vi "服务器引用层次.vi"(1 "服务器引用层次 i":T1, 2 "模式":enum16{"读取", "写入"}(ring)) -> (0 "服务器引用层次 o":T1)   [LabVIEW 2013]
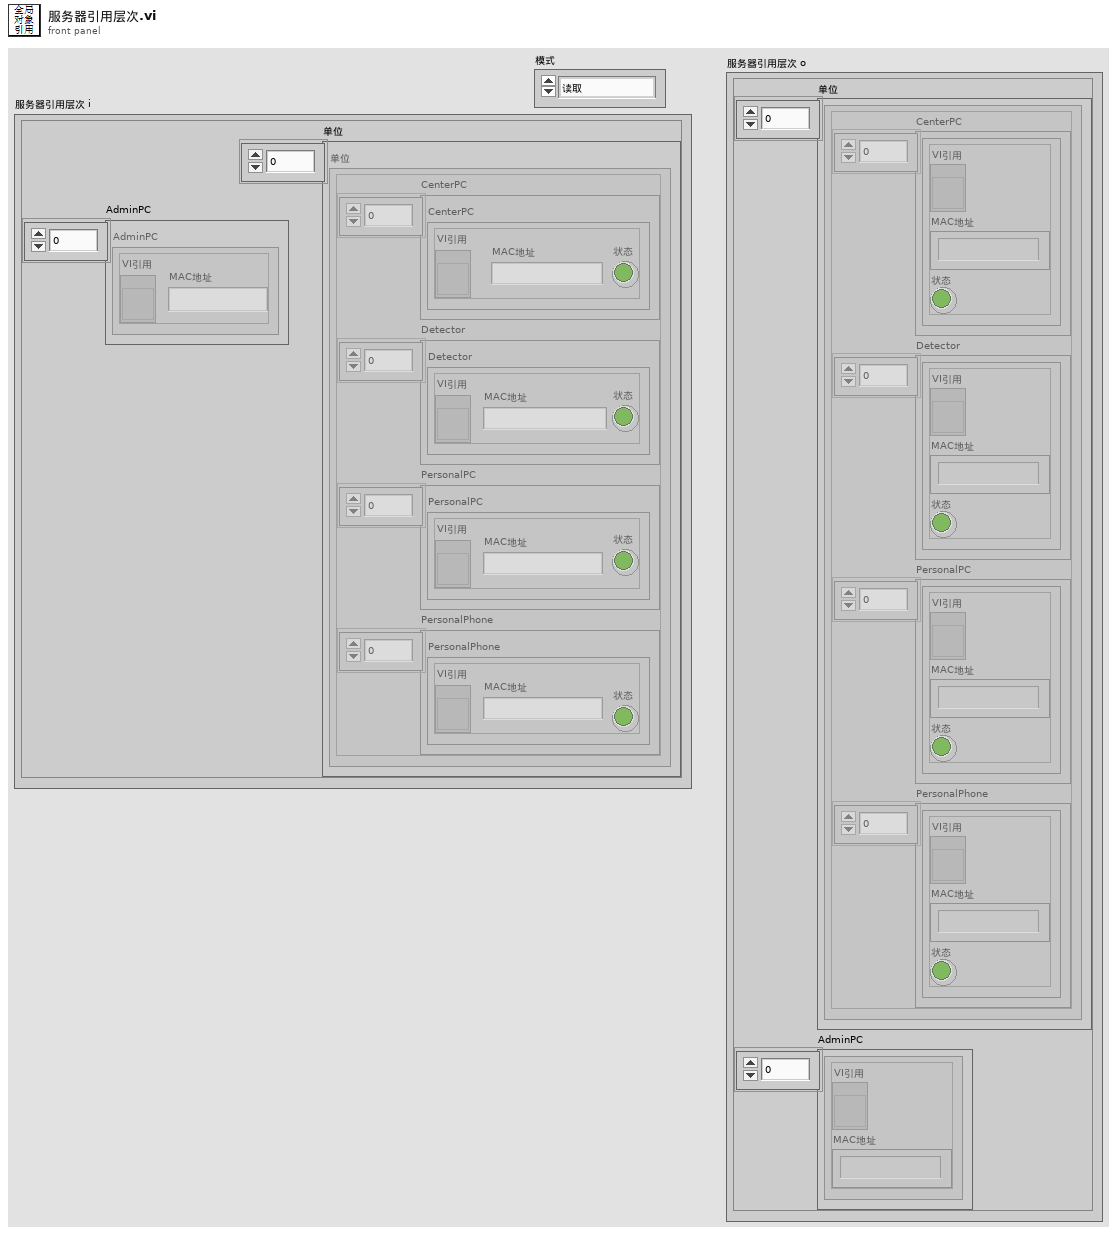
[diagram p1: front panel]
types:
  T1 = cluster{"单位":cluster{"CenterPC":cluster{"VI引用":refnum<vi>, "MAC地址":string, "状态":bool}[], "Detector":cluster{"VI引用":refnum<vi>, "MAC地址":string, "状态":bool}[], "PersonalPC":cluster{"VI引用":refnum<vi>, "MAC地址":string, "状态":bool}[], "PersonalPhone":cluster{"VI引用":refnum<vi>, "MAC地址":string, "状态":bool}[]}[], "AdminPC":cluster{"VI引用":refnum<vi>, "MAC地址":string}[]}
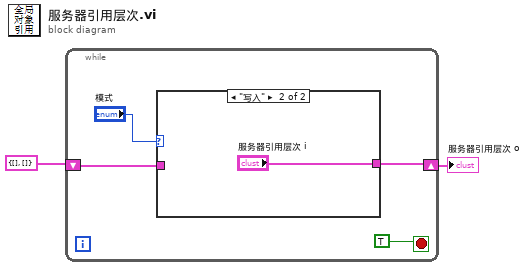
[diagram p0: block diagram]
diagram:
  n1 = while {
    shift-right: [w4] -> w1
    shift-left: T1 {"单位"=[], "AdminPC"=[]} ("服务器引用层次") -> [w3]
    stop <- TRUE stop-if-true
    n2 = case shown="\"写入\"" "模式" {
      tunnel: [w7 "服务器引用层次 i"] -> w4
      tunnel: w3 -> [w7 _]
      frame "读取", Default {
      }
      frame "写入" {
      }
    }
  }
  "服务器引用层次 o" <- w1
